vi "Finish.vi"   [LabVIEW 2023]
doc: "This VI is called just before exiting. It is expected to close I/O refnum, save collected data, etc."
uses:
  <vilib>/Rock Robotics/WPI/Utilities/WPI_GetSetVariantRefNum.vi
types:
  T1 = typedef "WPI_RobotDriveDevRef.ctl" = cluster{"DevStatus":errorcluster, "Motors[]":T2[], "Square Inputs":bool, "Max Output":dbl}
  T2 = typedef "WPI_MotorControlDeviceRef.ctl" = cluster{"DeviceStatus":errorcluster, "Type":T3, "PWM":cluster{"PWM Channel":T4, "DeadBand":T5}, "CAN":cluster{"Device Number":u8, "SetOutput VI Ref":variant, "GetOutput VI Ref":variant, "Enable VI Ref":variant, "Disable VI Ref":variant, "Data":variant}, "Invert":bool, "DIO PWM":cluster{"PWM \"Enable\" Channel":T4, "DIOChannel":T6, "PWM Rate":dbl}}
  T3 = typedef "WPI_MotorControlType.ctl" = enum16{"PWM", "CAN", "DIO PWM"}
  T4 = typedef "FPGA_DIOPWMChannel.ctl" = enum8{"PWM 0", "PWM 1", "PWM 2", "PWM 3", "PWM 4", "PWM 5", "PWM 6", "PWM 7", "PWM 8", "PWM 9", "PWM MXP 0", "PWM MXP 1", "PWM MXP 2", "PWM MXP 3", "PWM MXP 4", "PWM MXP 5", "PWM MXP 6", "PWM MXP 7", "PWM MXP 8", "PWM MXP 9", "Invalid"}
  T5 = typedef "WPI_PWMDeadband.ctl" = cluster{"Name":string, "maxPositivePwm":i32, "minPositivePwm":i32, "centerPwm":i32, "maxNegativePwm":i32, "minNegativePwm":i32, "angularRange":u16}
  T6 = typedef "FPGA_DIOChannel.ctl" = enum8{"DIO 0", "DIO 1", "DIO 2", "DIO 3", "DIO 4", "DIO 5", "DIO 6", "DIO 7", "DIO 8", "DIO 9", "DIO MXP 0", "DIO MXP 1", "DIO MXP 2", "DIO MXP 3", "DIO MXP 4", "DIO MXP 5", "DIO MXP 6", "DIO MXP 7", "DIO MXP 8", "DIO MXP 9", "DIO MXP 10", "DIO MXP 11", "DIO MXP 12", "DIO MXP 13", "DIO MXP 14", "DIO MXP 15", "SPI Port CS1", "SPI Port CS2", "SPI Port CS3", "SPI Port MISO", "SPI Port MOSI", "Invalid"}
  T7 = typedef "WPI_JoystickDevRef.ctl" = cluster{"Device":T8}
  T8 = typedef "WPI_JoystickDeviceEnum.ctl" = enum16{"USB 0", "USB 1", "USB 2", "USB 3", "USB 4", "USB 5"}
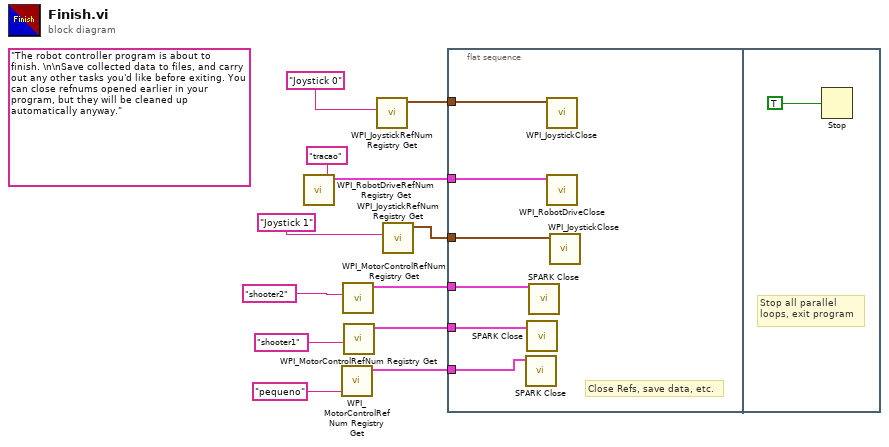
[diagram p0: block diagram]
diagram:
  (unwired) "The robot controller program is about to finish. \n\nSave collected data to files, and carry out any other tasks you'd like before exiting. You can close refnums opened earlier in your program, but they will be cleaned up automatically anyway."
  n1 = call <vilib>:"WPI_RobotDriveRefNum Registry Get.vi"("refnum name"="tracao") -> ("RobotDriveDevRef"=w10:T1)  [unwired: 1 in, 9 out]
  n2 = call <vilib>:"WPI_MotorControlRefNum Registry Get.vi"("refnum name"="pequeno") -> ("MotorControlDevRef"=w1:T2)  [unwired: 9 in, 1 out]
  n3 = call <vilib>:"WPI_MotorControlRefNum Registry Get.vi"("refnum name"="shooter2") -> ("MotorControlDevRef"=w3:T2)  [unwired: 9 in, 1 out]
  n4 = call <vilib>:"WPI_MotorControlRefNum Registry Get.vi"("refnum name"="shooter1") -> ("MotorControlDevRef"=w2:T2)  [unwired: 9 in, 1 out]
  n5 = call <vilib>:"WPI_JoystickRefNum Registry Get.vi"("refnum name"="Joystick 0") -> ("JoystickDevRef"=w9:T7)  [unwired: 1 in, 9 out]
  n6 = call <vilib>:"WPI_JoystickRefNum Registry Get.vi"("refnum name"="Joystick 1") -> ("JoystickDevRef"=w7:T7)  [unwired: 1 in, 9 out]
  n7 = flat-sequence {
    tunnel: w10 -> [w18]
    tunnel: w9 -> [w17]
    tunnel: w7 -> [w16]
    tunnel: w3 -> [w15]
    tunnel: w2 -> [w14]
    tunnel: w1 -> [w13]
    frame #0 {
      # "Close Refs, save data, etc."
      n8 = call <vilib>:"SPARK Close.vi"("MotorControlDeviceRef"=w13) -> ()  [unwired: 10 in, 1 out]
      n9 = call <vilib>:"SPARK Close.vi"("MotorControlDeviceRef"=w14) -> ()  [unwired: 10 in, 1 out]
      n10 = call <vilib>:"SPARK Close.vi"("MotorControlDeviceRef"=w15) -> ()  [unwired: 10 in, 1 out]
      n11 = call <vilib>:"WPI_JoystickClose.vi"("JoystickDevRef"=w17) -> ()  [unwired: 11 out]
      n12 = call <vilib>:"WPI_RobotDriveClose.vi"("RobotDriveDevRef"=w18) -> ()  [unwired: 1 in, 10 out]
      n13 = call <vilib>:"WPI_JoystickClose.vi"("JoystickDevRef"=w16) -> ()  [unwired: 11 out]
    }
    frame #1 {
      # "Stop all parallel\nloops, exit program"
      n14 = Stop(stop? (T)=TRUE ("Quit")) -> ()
    }
  }
